vi "Practica 5.vi"() -> ()   [LabVIEW 2020]
uses:
  <vilib>/addons/control/pid/pid.llb/PID (DBL).vi
  <vilib>/addons/control/pid/NI_PID_pid.lvlib
panel:
  in  "stop":bool
  out "Waveform Chart":dynamicdata(graph)
  in  "Slide":dbl(slide) scale=0.0..5.0
  in  "PID gains":T1={"proportional gain (Kc)"=1.0, "integral time (Ti, min)"=0.01, "derivative time (Td, min)"=0.0} {"derivative time (Td, min)" format="%.3f"; "integral time (Ti, min)" format="%.3f"; "proportional gain (Kc)" format="%.3f"}
  in  "output range":cluster{"output high":dbl, "output low":dbl}={"output high"=100.0, "output low"=-100.0} {"output low" format="%.2f"; "output high" format="%.2f"}
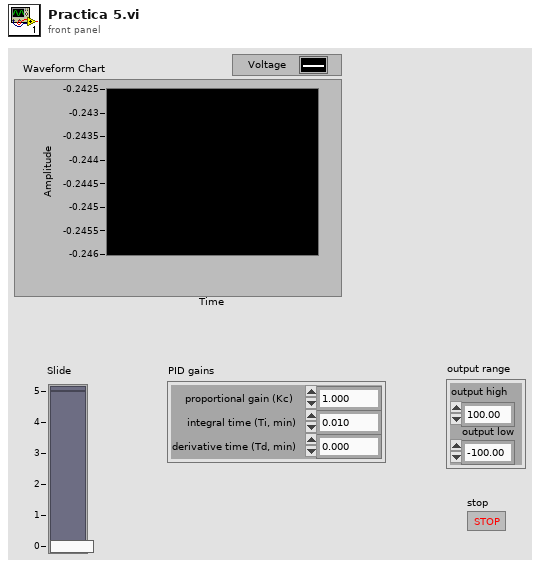
[diagram p1: front panel]
types:
  T1 = cluster{"proportional gain (Kc)":dbl, "integral time (Ti, min)":dbl, "derivative time (Td, min)":dbl}
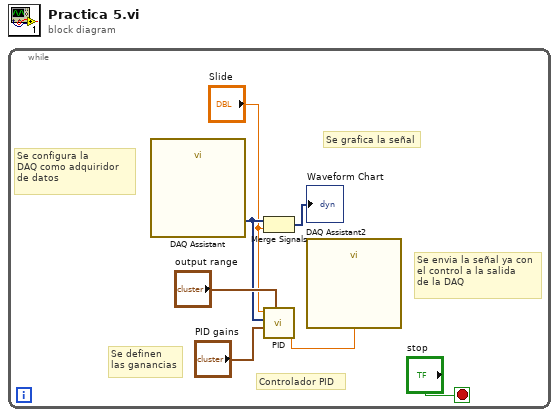
[diagram p0: block diagram]
diagram:
  n1 = while {
    stop <- "stop" stop-if-true
    # "Controlador PID"
    # "Se grafica la señal"
    # "Se envia la señal ya con\nel control a la salida\nde la DAQ"
    # "Se definen \nlas ganancias"
    # "Se configura la \nDAQ como adquiridor\nde datos"
    n2 = call "DAQ Assistant"() -> ("data"=w2:dynamicdata)  [unwired: 17 in, 2 out]
    n3 = Merge Signals(w2, "Slide") -> (→"Waveform Chart":dynamicdata)
    n4 = call-poly <vilib>:"PID.vi"("output range"="output range", "PID gains"="PID gains", "process variable"=w2, "setpoint"="Slide") -> ("output"=w4:dbl)  [unwired: 6 in, 1 out]
    n5 = call "DAQ Assistant2"("data"=w4) -> ()  [unwired: 17 in, 2 out]
  }
